vi "Destroy_user_event.vi"(11 "Test_Caller in":refnum<class "Test_Caller.lvclass">) -> (0 "error out":errorcluster, 3 "Test_Caller out":refnum<class "Test_Caller.lvclass">)   [LabVIEW 2025, in "Test_Caller.lvlib" / "Test_Caller.lvclass"]
uses:
  Test_Caller.lvclass
  Test_Caller.lvclass/Test_Caller.ctl
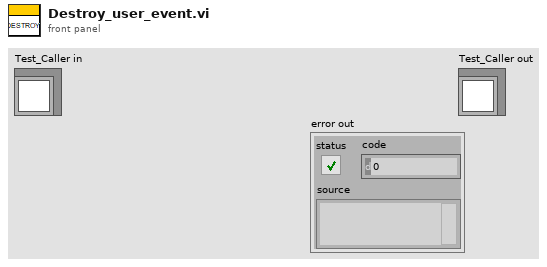
[diagram p1: front panel]
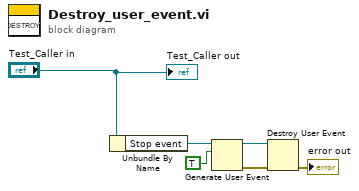
[diagram p0: block diagram]
diagram:
  n1 = Unbundle By Name("Test_Caller in") -> ("Stop event"=w5:refnum<user-event>)
  n2 = Generate User Event(user event=w5, event data cluster=TRUE ("event data")) -> (user event out=w2:refnum<user-event>, error out=w3:errorcluster)  [unwired: 2 in]
  n3 = Destroy User Event(user event=w2, error in=w3) -> (error out=→"error out":errorcluster)
  "Test_Caller out" <- "Test_Caller in"
